vi "Config IQ Skew Correction.vi"(0 "VISA Resource Name":refnum<visa-resource-name>, 5 "State (T: ON)":bool=TRUE, 7 "Skew Path  (0: RF)":enum16{"RF", "BB"}(ring) format="%.0g", 9 "Skew (0.0)":dbl, 11 "error in (no error)":errorcluster {"code" format="%.0x"}) -> (4 "VISA Resource Name Out":refnum<visa-resource-name>, 15 "error out":errorcluster {"code" format="%.0x"})   [LabVIEW 2014, in "Agilent ESG Series.lvlib"]
doc: "This VI configures alternate amplitude.\n\nNotes:\n(1) This VI is supported for Agilent 44xxB with option UNA or Agilent E4438C only."
uses:
  Agilent ESG Series.lvlib
panel:
  # "ON"
  # "OFF"
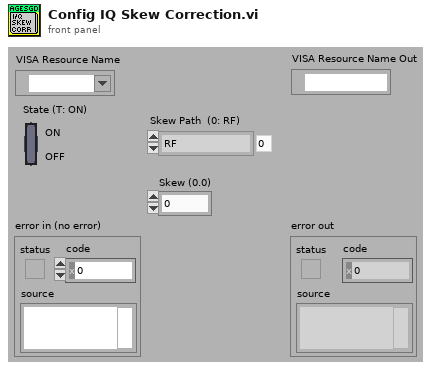
[diagram p1: front panel]
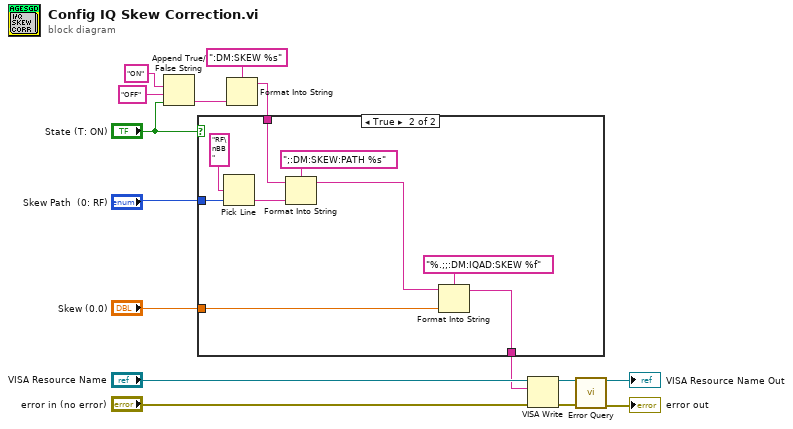
[diagram p0: block diagram]
diagram:
  n1 = Append True/False String(1:"State (T: ON)", 2:"OFF" ("false string"), 3:"ON" ("multi-line string")) -> (0:w4:string)  [unwired: 1 in]
  n2 = Format Into String(format string=":DM:SKEW %s", w4) -> (resulting string=w5:string)  [unwired: 2 in, 1 out]
  n3 = case shown="True" "State (T: ON)" {
    tunnel: "Skew Path  (0: RF)" -> [_ w22]
    tunnel: "Skew (0.0)" -> [_ w21]
    tunnel: w5 -> [w16 w20]
    tunnel: [w16 w18] -> w1
    frame False {
    }
    frame True {
      n4 = Pick Line(multi-line string="RF\nBB", line index=w22) -> (output string=w25:string)  [unwired: 1 in]
      n5 = Format Into String(format string=";:DM:SKEW:PATH %s", initial string=w20, w25) -> (resulting string=w19:string)  [unwired: 1 in, 1 out]
      n6 = Format Into String(format string="%.;;:DM:IQAD:SKEW %f", initial string=w19, w21) -> (resulting string=w18:string)  [unwired: 1 in, 1 out]
    }
  }
  n7 = VISA Write(VISA resource name="VISA Resource Name", write buffer=w1, error in (no error)="error in (no error)") -> (VISA resource name out=w11:refnum<visa-resource-name>, error out=w10:errorcluster)  [unwired: 1 out]
  n8 = call "Error Query.vi"("VISA Resource Name"=w11, "error in (no error)"=w10) -> ("VISA Resource Name Out"=→"VISA Resource Name Out":refnum<visa-resource-name>, "error out"=→"error out":errorcluster)  [unwired: 10 in, 2 out]
